vi "Update Buttons.vi"(8 "error in (no error)":errorcluster, 9 "Button State":T2=enum."No Next", 10 "Execution State in":T1=enum."Idle", 11 "Ctl Refs in":T3) -> (0 "error out":errorcluster, 2 "Execution State out":T1=enum."Idle", 3 "Ctl Refs out":T3)   [LabVIEW 2013]
uses:
  Controls/Refs.ctl
  Controls/Button Refs.ctl
  Controls/Tab Ctl Refs.ctl
  types/TabStateType.ctl
  Controls/Indicator Refs.ctl
  Controls/Slider Refs.ctl
  Controls/Control Refs.ctl
  types/ButtonStateType.ctl
  types/ExecutionStateType.ctl
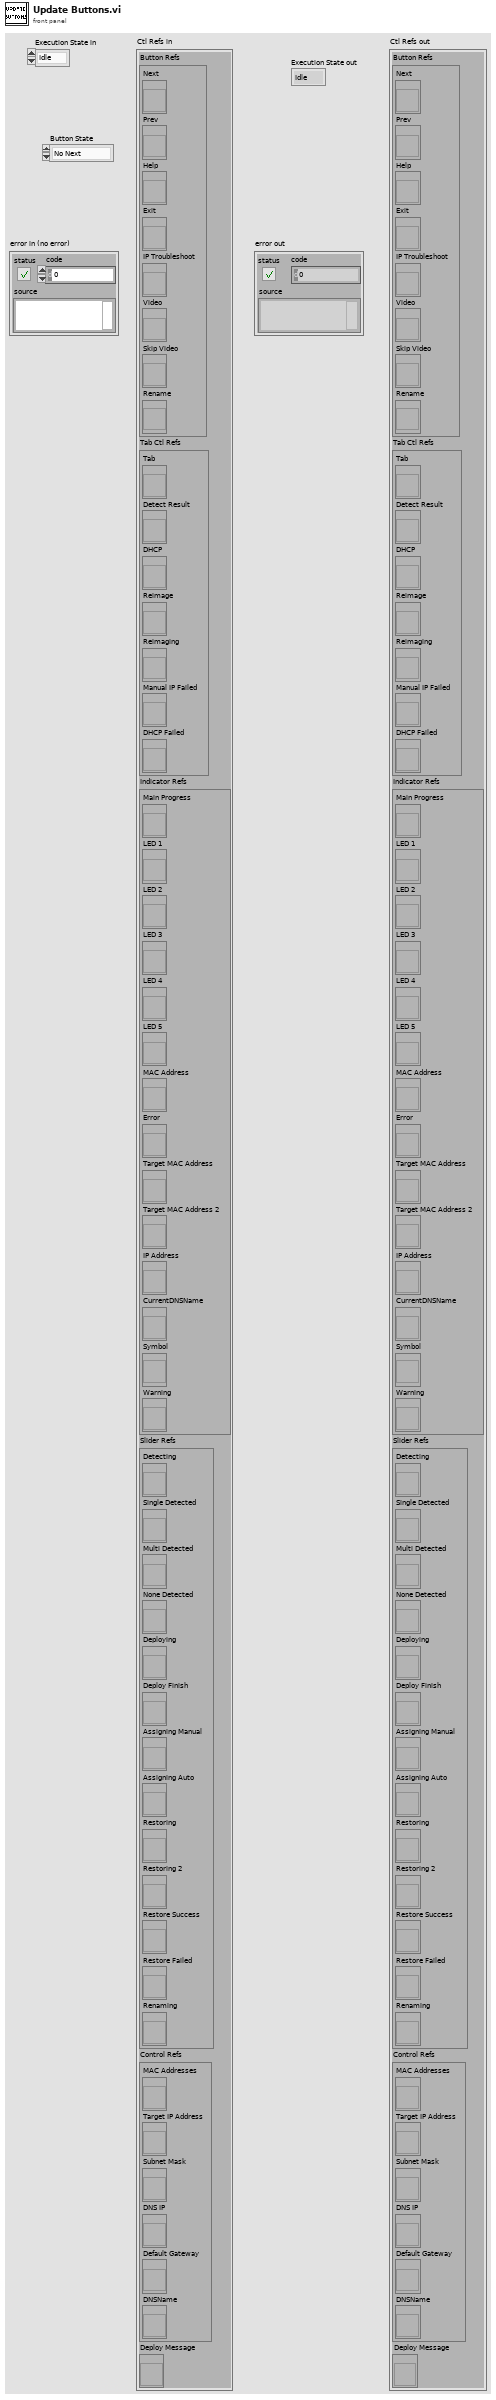
[diagram p1: front panel]
types:
  T1 = typedef "ExecutionStateType.ctl" = enum16{"Init", "Welcome", "Idle", "Detect", "Run Detection", "Detect Fail", "Detect One", "Detect Mult", "Deploy", "DHCP", "Static IP", "Run Deployment", "Connect Verify", "Exit", "Video Wait", "Success", "Troubleshoot", "Troubleshoot 2", "RenameDNS"}
  T2 = typedef "ButtonStateType.ctl" = enum16{"No change", "No Next", "No Prev", "All Disabled", "All Enabled", "Exit Only"}
  T3 = typedef "Refs.ctl" = cluster{"Button Refs":T4, "Tab Ctl Refs":T5, "Indicator Refs":T6, "Slider Refs":T7, "Control Refs":T8, "Deploy Message":refnum<vi>}
  T4 = typedef "Button Refs.ctl" = cluster{"Next":refnum<vi>, "Prev":refnum<vi>, "Help":refnum<vi>, "Exit":refnum<vi>, "IP Troubleshoot":refnum<vi>, "Video":refnum<vi>, "Skip Video":refnum<vi>, "Rename":refnum<vi>}
  T5 = typedef "Tab Ctl Refs.ctl" = cluster{"Tab":refnum<vi>, "Detect Result":refnum<vi>, "DHCP":refnum<vi>, "Reimage":refnum<vi>, "Reimaging":refnum<vi>, "Manual IP Failed":refnum<vi>, "DHCP Failed":refnum<vi>}
  T6 = typedef "Indicator Refs.ctl" = cluster{"Main Progress":refnum<vi>, "LED 1":refnum<vi>, "LED 2":refnum<vi>, "LED 3":refnum<vi>, "LED 4":refnum<vi>, "LED 5":refnum<vi>, "MAC Address":refnum<vi>, "Error":refnum<vi>, "Target MAC Address":refnum<vi>, "Target MAC Address 2":refnum<vi>, "IP Address":refnum<vi>, "CurrentDNSName":refnum<vi>, "Symbol":refnum<vi>, "Warning":refnum<vi>}
  T7 = typedef "Slider Refs.ctl" = cluster{"Detecting":refnum<vi>, "Single Detected":refnum<vi>, "Multi Detected":refnum<vi>, "None Detected":refnum<vi>, "Deploying":refnum<vi>, "Deploy Finish":refnum<vi>, "Assigning Manual":refnum<vi>, "Assigning Auto":refnum<vi>, "Restoring":refnum<vi>, "Restoring 2":refnum<vi>, "Restore Success":refnum<vi>, "Restore Failed":refnum<vi>, "Renaming":refnum<vi>}
  T8 = typedef "Control Refs.ctl" = cluster{"MAC Addresses":refnum<vi>, "Target IP Address":refnum<vi>, "Subnet Mask":refnum<vi>, "DNS IP":refnum<vi>, "Default Gateway":refnum<vi>, "DNSName":refnum<vi>}
  T9 = typedef "TabStateType.ctl" = enum32{"Welcome", "Instructions", "Detect", "Run Detection", "Detect Result", "Deploy", "Run Deployment", "Connect Verify", "Success", "DHCP", "Troubleshoot", "System Restore", "Error", "Video", "Rename"}
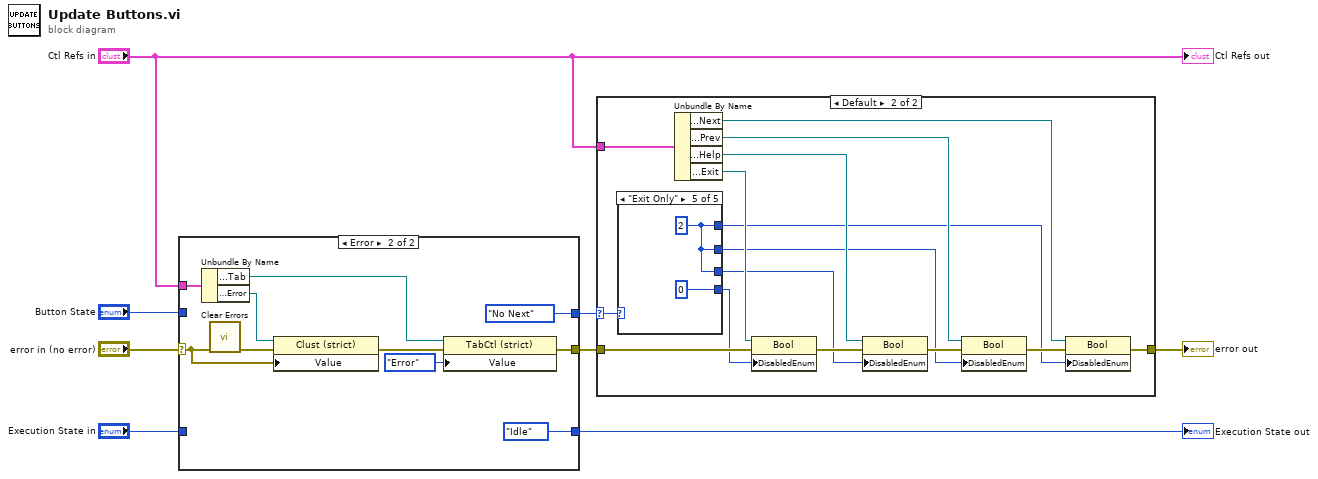
[diagram p0: block diagram]
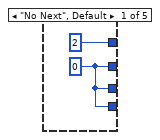
[diagram p3: hidden frame]
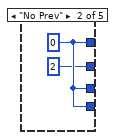
[diagram p4: hidden frame]
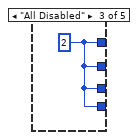
[diagram p5: hidden frame]
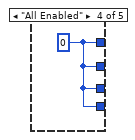
[diagram p6: hidden frame]
diagram:
  n1 = case shown="Error" "error in (no error)" {
    selector: "error in (no error)" -> [w9 w15]
    tunnel: "Button State" -> [w10 _]
    tunnel: "Ctl Refs in" -> [_ w19]
    tunnel: "Execution State in" -> [w11 _]
    tunnel: [w11 ExecutionStateType."Idle" ("Enum")] -> w1
    tunnel: [w10 ButtonStateType."No Next" ("Button State")] -> w4
    tunnel: [w9 w12] -> w3
    frame No Error {
    }
    frame Error {
      n2 = Unbundle By Name(w19) -> ("Tab Ctl Refs.Tab"=w18:refnum<vi>, "Indicator Refs.Error"=w16:refnum<vi>)
      n3 = call <vilib>:"Clear Errors.vi"("error in (no error)"=w15) -> ("error out"=w17:errorcluster)  [unwired: 6 out]
      n4 = property on="Property Node" class="Clust (strict)"(reference=w16, error in=w17, "Value"=w15) -> (error out=w14:errorcluster)  [unwired: 1 out]
      n5 = property on="Property Node" class="TabCtl (strict)"(reference=w18, error in=w14, "Value"=TabStateType."Error") -> (error out=w12:errorcluster)  [unwired: 1 out]
    }
  }
  "Execution State out" <- w1
  n6 = case shown="Default" w4 {
    selector: w4 -> [_ w28]
    tunnel: [w22 w36] -> w8
    tunnel: "Ctl Refs in" -> [_ w33]
    tunnel: w3 -> [w22 w27]
    frame "No change" {
    }
    frame Default {
      n7 = case shown="\"Exit Only\"" w28 {
        tunnel: [u8 2 ("Disabled") w41 w42 w43 w45] -> w23
        tunnel: [w39 u8 2 ("Disabled") w42 w43 w45] -> w24
        tunnel: [w39 w41 w42 w43 w45] -> w25
        tunnel: [w39 w41 w42 w43 u8 0 ("Disabled")] -> w26
        frame "No Next", Default {
          w39 = u8 0 ("Disabled")
        }
        frame "No Prev" {
          w41 = u8 0 ("Disabled")
        }
        frame "All Disabled" {
          w42 = u8 2 ("Disabled")
        }
        frame "All Enabled" {
          w43 = u8 0 ("Disabled")
        }
        frame "Exit Only" {
          w45 = u8 2 ("Disabled")
        }
      }
      n8 = Unbundle By Name(w33) -> ("Button Refs.Next"=w29:refnum<vi>, "Button Refs.Prev"=w30:refnum<vi>, "Button Refs.Help"=w31:refnum<vi>, "Button Refs.Exit"=w32:refnum<vi>)
      n9 = property class="Bool"(reference=w32, error in=w27, "DisabledEnum"=w26) -> (error out=w37:errorcluster)  [unwired: 1 out]
      n10 = property class="Bool"(reference=w31, error in=w37, "DisabledEnum"=w25) -> (error out=w34:errorcluster)  [unwired: 1 out]
      n11 = property class="Bool"(reference=w30, error in=w34, "DisabledEnum"=w24) -> (error out=w35:errorcluster)  [unwired: 1 out]
      n12 = property class="Bool"(reference=w29, error in=w35, "DisabledEnum"=w23) -> (error out=w36:errorcluster)  [unwired: 1 out]
    }
  }
  "error out" <- w8
  "Ctl Refs out" <- "Ctl Refs in"
